vi "Primary2Sorted.vi"(1 "Primary channel coincidences":T2[](array[typedef])) -> (0 "Sorted data":T1(array[cluster]))   [LabVIEW 2016]
uses:
  Typedefs/Coincidence.ctl
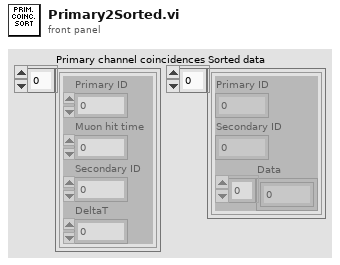
[diagram p1: front panel]
types:
  T1 = cluster{"Primary ID":i8, "Secondary ID":i8, "Data":i32[]}[]
  T2 = typedef "Coincidence.ctl" = cluster{"Primary ID":i8, "Muon hit time":u64, "Secondary ID":i8, "DeltaT":i32}
  T3 = cluster{"Primary ID":i8, "Secondary ID":i8, "Data":i32[]}
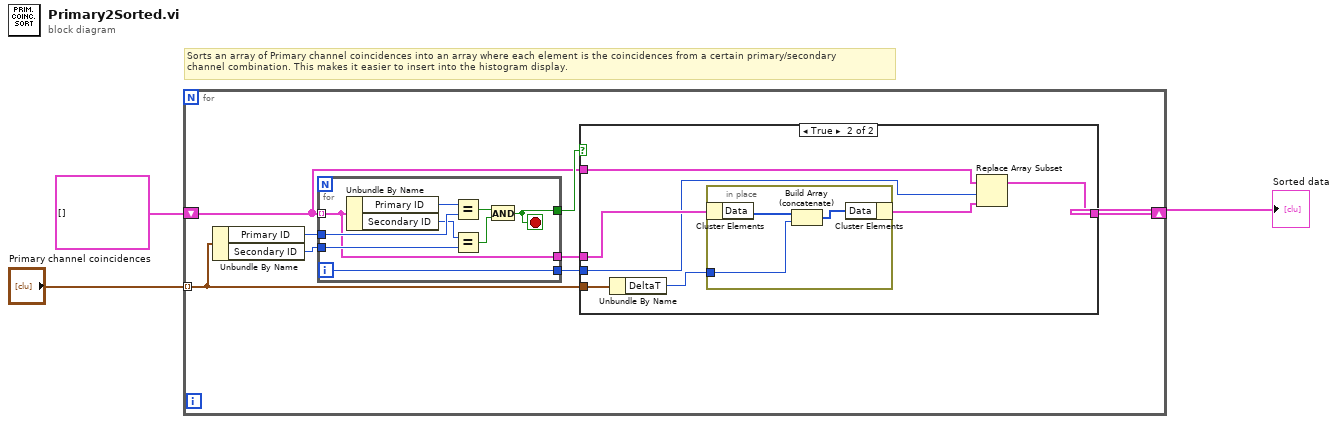
[diagram p0: block diagram]
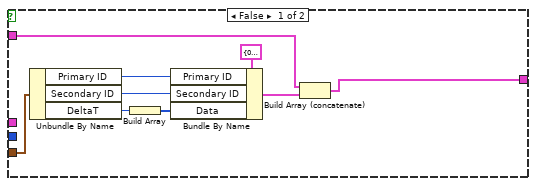
[diagram p2: hidden frame]
diagram:
  # "Sorts an array of Primary channel coincidences into an array where each element is the coincidences from a certain primary/secondary\nchannel combination. This makes it easier to insert into the histogram display."
  n1 = for {
    tunnel: "Primary channel coincidences" -> [w6] mode=indexing
    shift-right: [w7] -> w1
    shift-left: T1 [] ("Coincidence array") -> [w5]
    n2 = Unbundle By Name(w6) -> ("Primary ID"=w11:i8, "Secondary ID"=w10:i8)
    n3 = for {
      tunnel: w5 -> [w32] mode=indexing
      tunnel: w11 -> [w38]
      tunnel: w10 -> [w37]
      tunnel: [w33] -> w9
      tunnel: [w32] -> w8
      tunnel: [w31] -> w4
      i -> [w31]
      stop <- w33 stop-if-true
      n4 = Unbundle By Name(w32) -> ("Primary ID"=w39:i8, "Secondary ID"=w36:i8)
      n5 = Equal?(x=w39, y=w38) -> (x = y?=w34:bool)
      n6 = Equal?(x=w36, y=w37) -> (x = y?=w35:bool)
      n7 = And(x=w34, y=w35) -> (x .and. y?=w33:bool)
    }
    n8 = case shown="True" w9 {
      tunnel: w8 -> [_ w26]
      tunnel: [w16 w21] -> w7
      tunnel: w6 -> [w19 w27]
      tunnel: w5 -> [w14 w24]
      tunnel: w4 -> [_ w23]
      frame False {
        n9 = Unbundle By Name(w19) -> ("Primary ID"=w18:i8, "Secondary ID"=w17:i8, "DeltaT"=w13:i32)
        n10 = Build Array(w13) -> (w12:i32[])
        n11 = Bundle By Name(cluster=T3 {"Primary ID"=0, "Secondary ID"=0, "Data"=[]}, "Primary ID"=w18, "Secondary ID"=w17, "Data"=w12) -> (w15:T3)
        n12 = Build Array (concatenate)(w14, w15) -> (w16:T1)
      }
      frame True {
        n13 = Unbundle By Name(w27) -> ("DeltaT"=w25:i32)
        n14 = in-place {
          in-place-border: w25 -> [w29]
          n15 = in-place-cluster #1(w26) -> ("Data"=w30:i32[])
          n16 = Build Array (concatenate)(w30, w29) -> (w28:i32[])
          n17 = in-place-cluster #1("Data"=w28) -> (w22:T3)
        }
        n18 = Replace Array Subset(array=w24, new element=w22, index=w23) -> (w21:T1)
      }
    }
  }
  "Sorted data" <- w1
